vi "UDP receive.vi"(8 "error in":errorcluster, 10 "Timeout":i32=100, 11 "UDP connection ID":refnum<k16>) -> (0 "error out":errorcluster, 1 "Array01":dbl[](array[numeric]), 3 "UDP connection ID out":refnum<k16>, 4 "client port":u16, 6 "client IP address":string, 7 "raw data":string)   [LabVIEW 2018]
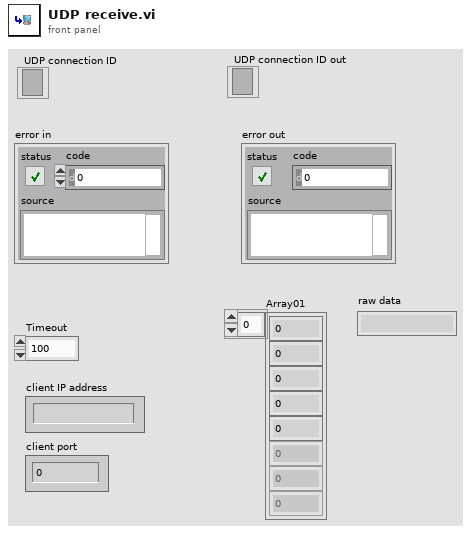
[diagram p1: front panel]
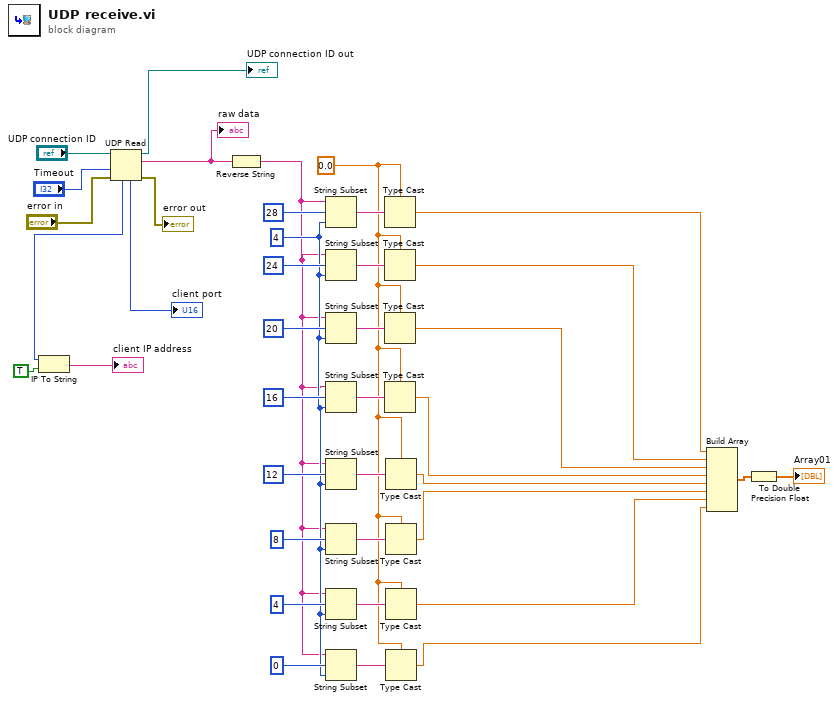
[diagram p0: block diagram]
diagram:
  w17 = 4 ("offset (0)")
  w16 = sgl 0.0
  n1 = UDP Read(connection ID="UDP connection ID", timeout ms (25000)="Timeout", 8:"error in") -> (data out=w10:string, error out=→"error out":errorcluster, 3:→"UDP connection ID out":refnum<k16>, 4:→"client port":u16, 6:w11:u32)  [unwired: 1 in]
  "raw data" <- w10
  n2 = IP To String(1:TRUE ("dot notation? (F)"), 2:w11) -> (0:→"client IP address":string)
  n3 = Reverse String(1:w10) -> (0:w15:string)
  n4 = String Subset(string=w15, offset (0)=28, length (rest)=w17) -> (substring=w18:string)
  n5 = String Subset(string=w15, offset (0)=24, length (rest)=w17) -> (substring=w21:string)
  n6 = String Subset(string=w15, offset (0)=20, length (rest)=w17) -> (substring=w23:string)
  n7 = String Subset(string=w15, offset (0)=16, length (rest)=w17) -> (substring=w25:string)
  n8 = String Subset(string=w15, offset (0)=12, length (rest)=w17) -> (substring=w37:string)
  n9 = String Subset(string=w15, offset (0)=8, length (rest)=w17) -> (substring=w38:string)
  n10 = String Subset(string=w15, offset (0)=4, length (rest)=w17) -> (substring=w39:string)
  n11 = String Subset(string=w15, offset (0)=0, length (rest)=w17) -> (substring=w33:string)
  n12 = Type Cast(type=w16, x=w18) -> (*(type *) &x=w8:sgl)
  n13 = Type Cast(type=w16, x=w21) -> (*(type *) &x=w7:sgl)
  n14 = Type Cast(type=w16, x=w23) -> (*(type *) &x=w6:sgl)
  n15 = Type Cast(type=w16, x=w25) -> (*(type *) &x=w5:sgl)
  n16 = Type Cast(type=w16, x=w37) -> (*(type *) &x=w4:sgl)
  n17 = Type Cast(type=w16, x=w38) -> (*(type *) &x=w3:sgl)
  n18 = Type Cast(type=w16, x=w39) -> (*(type *) &x=w2:sgl)
  n19 = Type Cast(type=w16, x=w33) -> (*(type *) &x=w1:sgl)
  n20 = Build Array(w8, w7, w6, w5, w4, w3, w2, w1) -> (w9:sgl[])
  n21 = To Double Precision Float(number=w9) -> (double precision float=→"Array01":dbl[])
